vi "create imaq user palettes.vi"(10 "max":dbl, 11 "palette":enum16{"EnhanceLow", "EnhanceLowMore", "Grey"}(ring)) -> (3 "Array":cluster{u8, "G":u8, u8}[](array[cluster]))   [LabVIEW 2013]
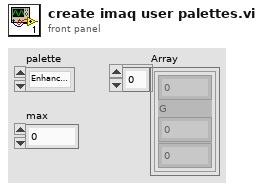
[diagram p1: front panel]
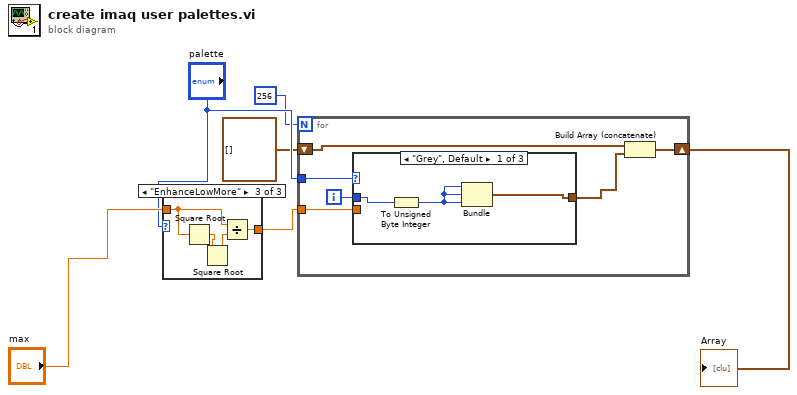
[diagram p0: block diagram]
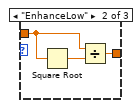
[diagram p3: hidden frame]
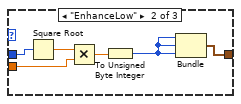
[diagram p4: hidden frame]
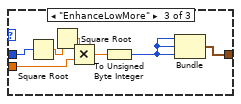
[diagram p5: hidden frame]
diagram:
  n1 = case shown="\"EnhanceLowMore\"" "palette" {
    tunnel: "max" -> [_ w8 w13]
    tunnel: [_ w7 w12] -> w4
    frame "Grey", Default {
    }
    frame "EnhanceLow" {
      n2 = Square Root(x=w8) -> (sqrt(x)=w9:dbl)
      n3 = Divide(x=w8, y=w9) -> (x/y=w7:dbl)
    }
    frame "EnhanceLowMore" {
      n4 = Square Root(x=w13) -> (sqrt(x)=w11:dbl)
      n5 = Square Root(x=w11) -> (sqrt(x)=w10:dbl)
      n6 = Divide(x=w13, y=w10) -> (x/y=w12:dbl)
    }
  }
  n7 = for {
    N: 256 -> [_]
    shift-right: [w18] -> w3
    shift-left: cluster{u8, "G":u8, u8}[] [] -> [w19]
    tunnel: w4 -> [w17]
    tunnel: "palette" -> [w16]
    i -> [w15]
    n8 = case shown="\"Grey\", Default" w16 {
      tunnel: w17 -> [_ w27 w35]
      tunnel: [w20 w23 w29] -> w14
      tunnel: w15 -> [w21 w26 w34]
      frame "Grey", Default {
        n9 = To Unsigned Byte Integer(number=w21) -> (unsigned 8bit integer=w22:u8)
        n10 = Bundle(w22, w22, w22) -> (w20:cluster{u8, u8, u8})  [unwired: 1 in]
      }
      frame "EnhanceLow" {
        n11 = Square Root(x=w26) -> (sqrt(x)=w28:dbl)
        n12 = Multiply(x=w28, y=w27) -> (x*y=w24:dbl)
        n13 = To Unsigned Byte Integer(number=w24) -> (unsigned 8bit integer=w25:u8)
        n14 = Bundle(w25, w25, w25) -> (w23:cluster{u8, u8, u8})  [unwired: 1 in]
      }
      frame "EnhanceLowMore" {
        n15 = Square Root(x=w34) -> (sqrt(x)=w33:dbl)
        n16 = Square Root(x=w33) -> (sqrt(x)=w32:dbl)
        n17 = Multiply(x=w32, y=w35) -> (x*y=w30:dbl)
        n18 = To Unsigned Byte Integer(number=w30) -> (unsigned 8bit integer=w31:u8)
        n19 = Bundle(w31, w31, w31) -> (w29:cluster{u8, u8, u8})  [unwired: 1 in]
      }
    }
    n20 = Build Array (concatenate)(w19, w14) -> (w18:cluster{u8, "G":u8, u8}[])
  }
  "Array" <- w3
